vi "Get elaphsd time for aiming.vi"(8 "Error in":errorcluster, 9 "Pause":bool, 10 "Reset":bool, 11 "Target time":dbl) -> (0 "Errorout":errorcluster, 1 "Elaphshed time":bool, 2 "Elaphsed time":dbl)   [LabVIEW 2020]
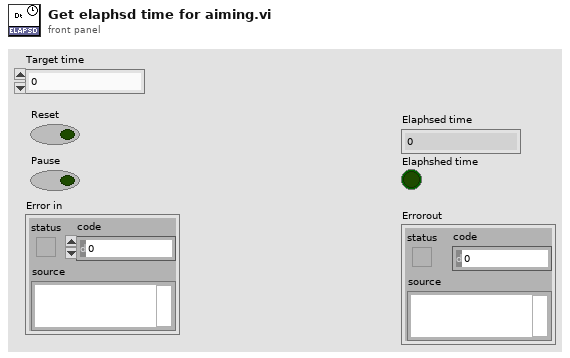
[diagram p1: front panel]
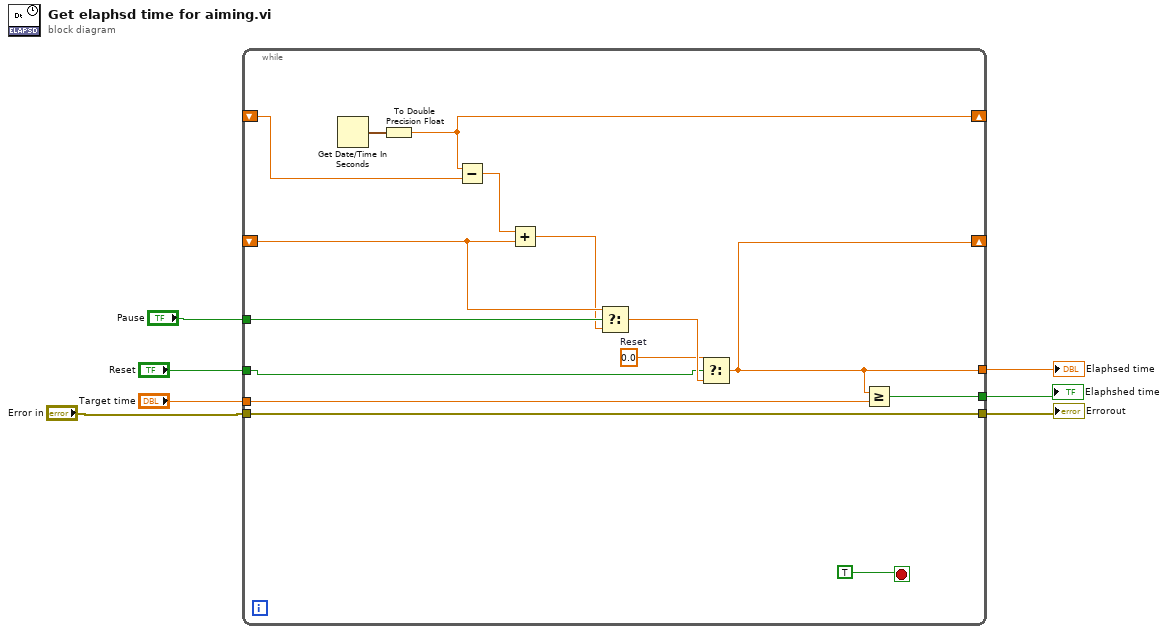
[diagram p0: block diagram]
diagram:
  n1 = while {
    shift-right: [w21] -> _
    shift-left: _ -> [w20]
    shift-right: [w11] -> _
    shift-left: _ -> [w17]
    tunnel: "Reset" -> [w8]
    tunnel: "Pause" -> [w18]
    tunnel: [w11] -> w5
    tunnel: [w13] -> w4
    tunnel: "Error in" -> [w13]
    tunnel: "Target time" -> [w12]
    tunnel: [w10] -> w2
    stop <- TRUE stop-if-true
    w14 = 0.0  # Reset
    n2 = Get Date/Time In Seconds() -> (seconds since 1Jan1904=w22:timestamp)
    n3 = To Double Precision Float(number=w22) -> (double precision float=w21:dbl)
    n4 = Subtract(x=w21, y=w20) -> (x-y=w19:dbl)
    n5 = Add(x=w19, y=w17) -> (x+y=w16:dbl)
    n6 = Select(t=w17, s=w18, f=w16) -> (s? t:f=w15:dbl)
    n7 = Select(t=w14, s=w8, f=w15) -> (s? t:f=w11:dbl)
    n8 = Greater Or Equal?(x=w11, y=w12) -> (x >= y?=w10:bool)
  }
  "Elaphsed time" <- w5
  "Errorout" <- w4
  "Elaphshed time" <- w2
